vi "GetDisplayForWindow.vi"(8 "No Error":errorcluster, 11 "Window [SDL_Window *]":T1 format="%.0x") -> (0 "Error Out":errorcluster, 3 "DisplayID":T2)   [LabVIEW 2026, in "SDL3.lvlib" / "Video.lvlib"]
doc: "<B>Summary</B>\nGet the display associated with a window."
uses:
  Video.lvlib
  DisplayID--integer.ctl
  <vilib>/Utility/error.llb/Error Cluster From Error Code.vi
  Error/Error.lvlib
  Lib/SDL3.dll
  SDL_Window--pointer.ctl
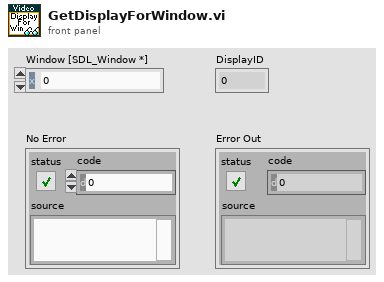
[diagram p1: front panel]
types:
  T1 = typedef "SDL3.lvlib/Video.lvlib/SDL_Window--pointer.ctl" = i64
  T2 = typedef "SDL3.lvlib/Video.lvlib/DisplayID--integer.ctl" = u32
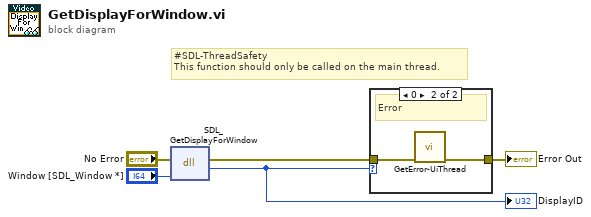
[diagram p0: block diagram]
diagram:
  # "#SDL-ThreadSafety\nThis function should only be called on the main thread."
  n1 = dll-call lib="C:/Users/saukko/Dev/LV-SDL3/Sources/SDL3/Lib/SDL3.*" fn="SDL_GetDisplayForWindow"(error in="No Error", "window"="Window [SDL_Window *]") -> (error out=w3:errorcluster, "return type"=w1:u32)  [unwired: 3 in, 1 out]
  "DisplayID" <- w1
  n2 = case shown="0" w1 {
    tunnel: w3 -> [w6 w8]
    tunnel: [w6 w7] -> w4
    frame Default {
      # "Ok"
    }
    frame 0 {
      # "Error"
      n3 = call "GetError-UiThread.vi"("No Error"=w8) -> ("error out"=w7:errorcluster)  [unwired: 10 in]
    }
  }
  "Error Out" <- w4
